vi "TCP Named Service - Server.vi"() -> ()   [LabVIEW 2014]
doc: "Creates a named service and listens on the first available port. When a client connects to the service, it sends a response string to the client."
panel:
  out "data out":string
  in  "Message to Send":string="You are currently accessing TCP Named Service - Server.vi from client %s on port %d."
  in  "Stop":bool
  # "Overview: Demonstrates the use of the TCP functions to initialize a named TCP service that can send data to a client VI.\nInstructions:\n1. Run the VI.\n2. Open TCP Named Service - Client.vi and follow the instructions on its front panel.\n3. Click Stop to stop the VI."
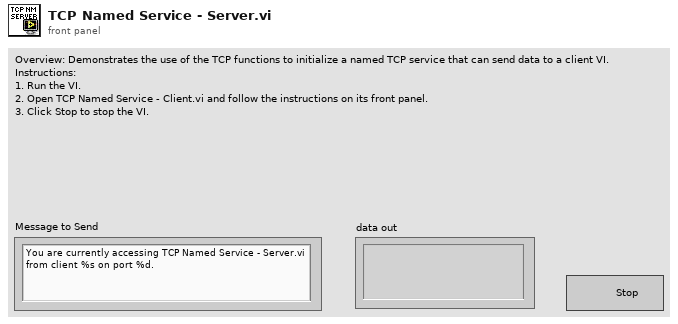
[diagram p1: front panel]
types:
  T1 = enum16{"Standard", "Buffered", "CRLF", "Immediate"}
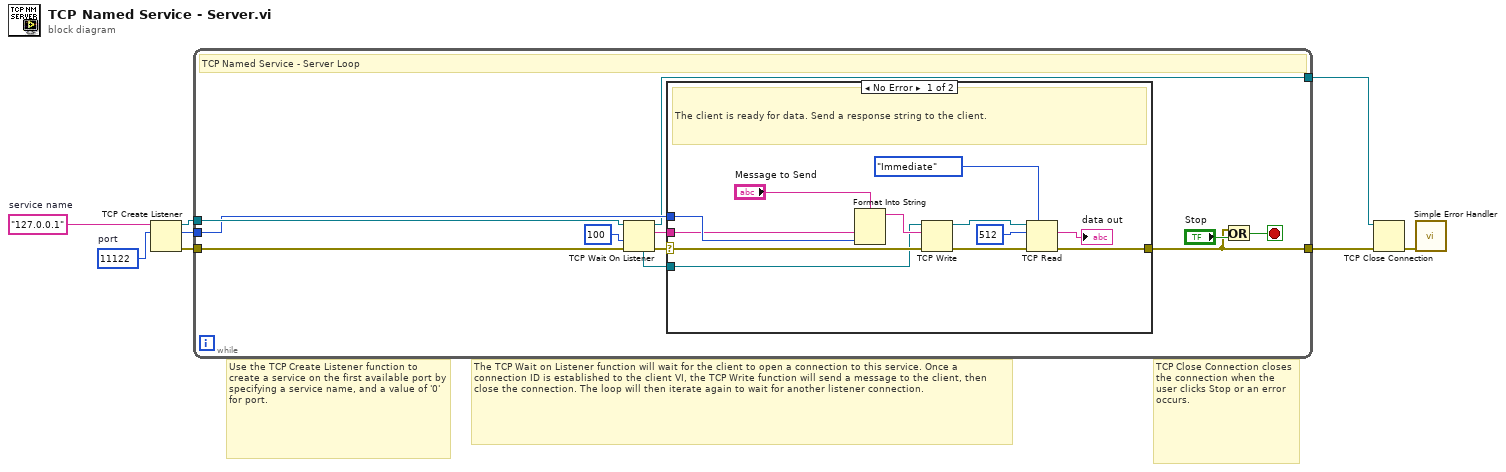
[diagram p0: block diagram]
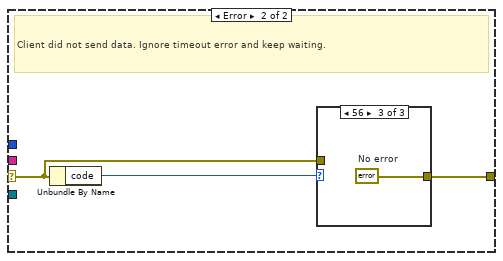
[diagram p2: hidden frame]
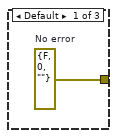
[diagram p3: hidden frame]
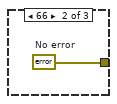
[diagram p4: hidden frame]
diagram:
  w3 = u16 11122  # port
  w2 = "127.0.0.1"  # service name
  # "TCP Close Connection closes the connection when the user clicks Stop or an error occurs."
  # "The TCP Wait on Listener function will wait for the client to open a connection to this service. Once a connection ID is established to the client VI, the TCP Write function will send a message to the client, then close the connection. The loop will then iterate again to wait for another listener connection."
  # "Use the TCP Create Listener function to create a service on the first available port by specifying a service name, and a value of '0' for port."
  n1 = TCP Create Listener(10:w3, 11:w2) -> (0:w7:errorcluster, 2:w5:u16, 3:w8:refnum<k5>)  [unwired: 3 in]
  n2 = while {
    tunnel: [w12] -> w1
    tunnel: w8 -> [w19]
    tunnel: w7 -> [w17]
    tunnel: [w9] -> w6
    tunnel: w5 -> [w15]
    stop <- w14 stop-if-true
    # "TCP Named Service - Server Loop"
    n3 = TCP Wait On Listener(8:w17, 9:100 ("timeout ms (25000)"), 11:w19) -> (0:w18:errorcluster, 2:w10:string, 3:w9:refnum<k5>, 4:w16:refnum<k5>)  [unwired: 1 in, 1 out]
    n4 = case shown="No Error" w18 {
      selector: w18 -> [w31 w34]
      tunnel: [w23 w32] -> w12
      tunnel: w16 -> [w26 _]
      tunnel: w15 -> [w30 _]
      tunnel: w10 -> [w28 _]
      frame No Error {
        # "The client is ready for data. Send a response string to the client."
        n5 = Format Into String(format string="Message to Send", w28, w30) -> (resulting string=w27:string)  [unwired: 2 in, 1 out]
        n6 = TCP Write(connection ID=w26, data in=w27, error in (no error)=w31) -> (connection ID out=w25:refnum<k5>, error out=w24:errorcluster)  [unwired: 1 in, 1 out]
        n7 = TCP Read(connection ID=w25, bytes to read=512, error in (no error)=w24, 7:T1."Immediate" ("mode (standard)")) -> (data out=→"data out":string, error out=w23:errorcluster)  [unwired: 1 in, 1 out]
      }
      frame Error {
        # "Client did not send data. Ignore timeout error and keep waiting."
        n8 = Unbundle By Name(w34) -> ("code"=w33:i32)
        n9 = case shown="56" w33 {
          tunnel: w34 -> [_ _ _]
          tunnel: [w35 w36 w37] -> w32
          frame Default {
            w35 = errorcluster {"status"=FALSE, "code"=0, "source"=""}  # No error
          }
          frame 66 {
            w36 = errorcluster {"status"=FALSE, "code"=0, "source"=""}  # No error
          }
          frame 56 {
            w37 = errorcluster {"status"=FALSE, "code"=0, "source"=""}  # No error
          }
        }
      }
    }
    n10 = Or(x=w12, y="Stop") -> (x .or. y?=w14:bool)
  }
  n11 = TCP Close Connection(connection ID=w6, error in (no error)=w1) -> (error out=w4:errorcluster)  [unwired: 1 in, 1 out]
  n12 = call <vilib>:"Simple Error Handler.vi"("error in (no error)"=w4) -> ()  [unwired: 4 in, 5 out]
